vi "RDV-togglePlotVisability.vi"(8 "error in (no error)":errorcluster, 11 "RDV-Reflection_Data_viewer in":refnum<class "RDV-Reflection_Data_viewer.lvclass">) -> (0 "error out":errorcluster, 3 "RDV-Reflection_Data_viewer out":refnum<class "RDV-Reflection_Data_viewer.lvclass">)   [LabVIEW 2020, in "RDV-Reflection_Data_viewer.lvclass"]
uses:
  RDV-Reflection_Data_viewer.lvclass
  RDV-Reflection_Data_viewer.lvclass/RDV-Reflection_Data_viewer.ctl
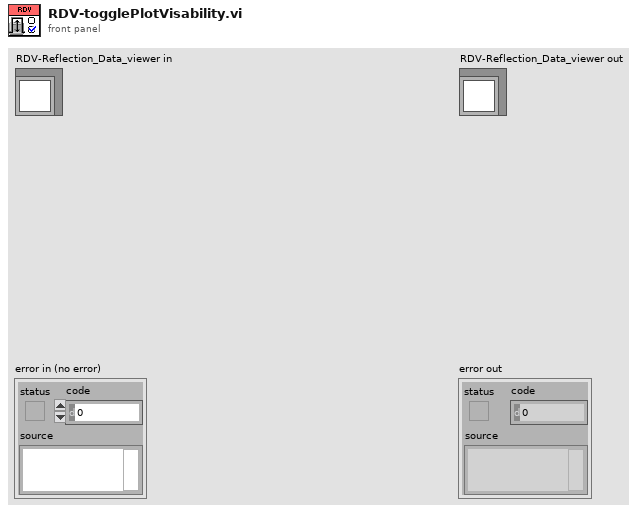
[diagram p1: front panel]
types:
  T1 = typedef "RDV-Reflection_Data_viewer.lvclass/RDV-XY_GRAPH_REFS.ctl" = cluster{"Reflection Real":refnum<vi>, "Reflection Imag":refnum<vi>, "Permittivity Real":refnum<vi>, "Permittivity Imag":refnum<vi>}
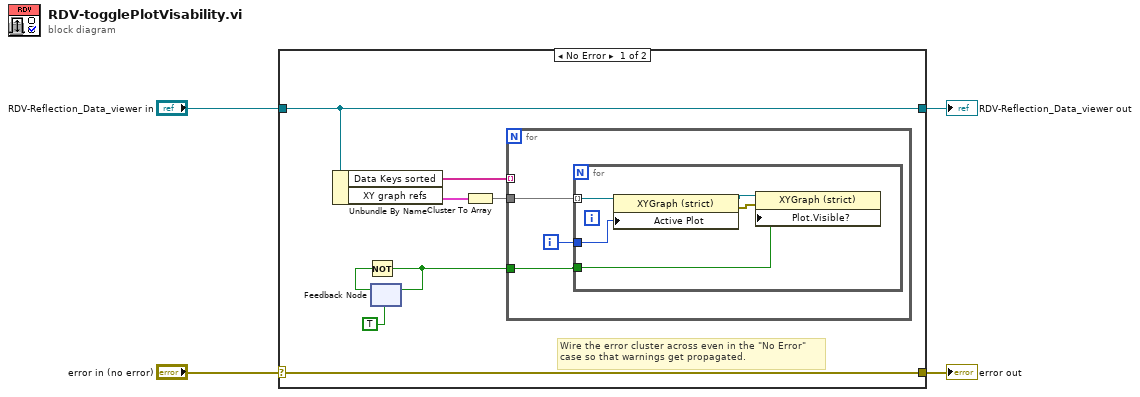
[diagram p0: block diagram]
diagram:
  n1 = case shown="No Error" "error in (no error)" {
    selector: "error in (no error)" -> [w12 w22]
    tunnel: [w12 w22] -> w3
    tunnel: [w9 w21] -> w1
    tunnel: "RDV-Reflection_Data_viewer in" -> [w9 w21]
    frame No Error {
      # "Wire the error cluster across even in the \"No Error\"\ncase so that warnings get propagated."
      n2 = Unbundle By Name(w9) -> ("Data Keys sorted"=w6:string[], "XY graph refs"=w7:T1)
      n3 = feedback #1(TRUE) -> (w10:bool)
      n4 = Not(x=w10) -> (.not. x?=w8:bool)
      n5 = feedback-in #1(w8) -> ()
      n6 = Cluster To Array(cluster=w7) -> (array=w5:refnum<vi>[])
      n7 = for {
        tunnel: w8 -> [w15]
        tunnel: w5 -> [w14]
        tunnel: w6 -> [_] mode=indexing
        i -> [w13]
        n8 = for {
          tunnel: w15 -> [w20]
          tunnel: w14 -> [w19] mode=indexing
          tunnel: w13 -> [w16]
          n9 = property on="Property Node" class="XYGraph (strict)"(reference=w19, "Active Plot"=w16) -> (reference out=w18:refnum<vi>, error out=w17:errorcluster)  [unwired: 1 in]
          n10 = property on="Property Node" class="XYGraph (strict)"(reference=w18, error in=w17, "Plot.Visible?"=w20) -> ()  [unwired: 2 out]
        }
      }
    }
    frame Error {
    }
  }
  "error out" <- w3
  "RDV-Reflection_Data_viewer out" <- w1
